vi "RF Streaming to Disk (Host).vi"() -> ()   [LabVIEW 2018]
doc: "This template is for the Simple NI-USRP Streaming design, a design that shows the basics of streaming data to and from an NI USRP-294x/295x device. Refer to the block diagram for more information about how to use this template."
uses:
  <vilib>/userdefined/Silver/nirio_resource_slv.ctl
  typedefs/rx channel config.ctl
  typedefs/rf.channel selector.ctl
  <vilib>/Utility/error.llb/DialogType.ctl
  typedefs/rx config.ctl
  SubVIs/RF Rec Start Trigger.ctl
panel:
  out "size (in bytes)":i64
  out "fifo fullness":dbl(slide) scale=0.0..1.0
  out "HW stoped":bool
  in  "Rec file":path=path "C:/Users/PLM_410/Загрузки/RF Recorder test.bin"
  in  "rf channel selector":T1
  in  "rx channel config":T2={"antenna"="RX2", "frequency"=2000000000.0, "lo frequency"=-1.0, "level"=0.0} {"frequency" format="%#.3pHz"; "lo frequency" format="%#.3pHz"; "level" format="%#_gdBm"}
  in  "number of samples":u32=8192 caption="Number of Samples"
  in  "sample rate":dbl=10000000.0 caption="Sample Rate" format="%#.3pS/s"
  in  "transfer mode":enum16{"Finite", "Continuous"}(ring) caption="Acquisition Mode"
  in  "USRP RIO device":T3="MXI1Port1Dev1" caption="USRP RIO Device"
  in  "indicator tab":T4(tab)
  out "power spectrum":cluster{"f0":dbl, "df":dbl, "magnitude":dbl[]}(graph) caption="Power Spectrum"
  out "power level":dbl[](graph) caption="Power Level"
  out "iq data":waveform(dbl)[](graph) caption="I & Q Data"
  out "rx.coerced configurations":T5 {"coerced sample rates" format="%#.3pS/s"; "coerced levels" format="%#.3gdBm"; "coerced lo frequencies" format="%#.3pHz"; "coerced frequencies" format="%#.3pHz"}
  in  "rx.stop":bool
  # "NI-USRP RIO Streaming to Disk"
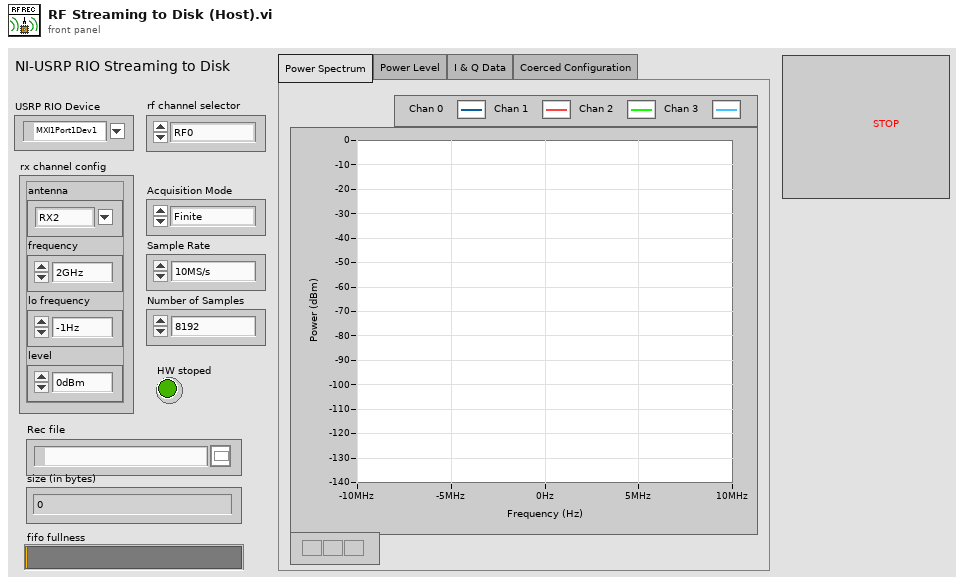
[diagram p1: front panel]
types:
  T1 = typedef "rf.channel selector.ctl" = enum16{"RF0", "RF1"}
  T2 = typedef "rx channel config.ctl" = cluster{"antenna":string, "frequency":dbl, "lo frequency":dbl, "level":dbl}
  T3 = typedef "nirio_resource_slv.ctl" = tag
  T4 = enum32{"Power Spectrum", "Power Level", "I & Q Data", "Coerced Configuration"}
  T5 = cluster{"coerced frequencies":dbl[], "coerced lo frequencies":dbl[], "coerced levels":dbl[], "coerced sample rates":dbl[]}
  T6 = enum16{"open", "replace", "create", "open or create", "replace or create", "replace or create with confirmation"}
  T7 = typedef "RF Rec Start Trigger.ctl" = enum8{"Software", "Digital Edge", "Rx Start Trigger", "Tx Start Trigger", "Immediate", "Future Time Event"}
  T8 = typedef "rx config.ctl" = cluster{"rf enable 0":bool, "rf config 0":cluster{"antenna":string, "frequency":dbl, "lo frequency":dbl, "level":dbl}, "rf enable 1":bool, "rf config 1":cluster{"antenna":string, "frequency":dbl, "lo frequency":dbl, "level":dbl}, "transfer mode":enum16{"Finite", "Continuous"}, "sample rate":dbl, "number of samples":u32, "start trigger":T7}
  T9 = cluster{"daughterboard 0 lo configuration":enum16{"Independent", "Import", "Shared and Export", "Reimport", "Shared"}, "daughterboard 1 lo configuration":enum16{"Independent", "Import", "Shared and Export", "Reimport", "Shared"}}
  T10 = typedef "DialogType.ctl" = u16
  T11 = typedef "niUsrpRio Config v1 Host.lvlib/niUsrpRio Session.ctl" = cluster{"FPGA Interface":refnum<k20>, "RIO Interface Number":u32, "Data Clock Rate":u32, "FPGA Data Clock Rate":u32, "Global Settings Register Bus":T12, "Radio 0 Settings Register Bus":T12, "Radio 1 Settings Register Bus":T12, "Radio Settings Bus Semaphore":T13, "DB Queues":T14[], "Characterization Data Valid?":bool, "EEPROM Header":T15, "Device Data Header":T16, "EEPROM Characterization Header":T17, "Characterization Data":T18[], "FPGA Current Version":u32, "FPGA Oldest Compatible Version":u32, "Fixed Logic Current Version":u32, "Fixed Logic Oldest Compatible Version":u32, "FPGA Radio Settings Bus Current Version":u32, "FPGA Radio Settings Bus Oldest Compatible Version":u32, "FPGA Board Config Current Version":u32, "FPGA Board Config Oldest Compatible Version":u32, "Daughterboard Clock Rate":u32, "daughterboard configuration session handles":u64[]}
  T12 = typedef "niInstr Register Bus v0 Host.lvlib/Register Bus Session.ctl" = refnum<queue>
  T13 = typedef "Semaphore RefNum" = refnum<k1>
  T14 = typedef "niUsrpRio Config v1 Host.lvlib/DB Queue Reference.ctl" = refnum<queue>
  T15 = typedef "niUsrpRio Config v1 Host.lvlib/EEPROM Header.ctl" = cluster{"Checksum":u32, "Product Code":u16, "Hardware Current Version":u16, "Hardware Oldest Compatible Version":u16, "EEPROM Map Current Version":u16, "EEPROM Map Oldest Compatible Version":u16, "User Password":string, "Pointer to Factory Header":u32, "Pointer to User Header":u32, "Recommended Interval":u16, "Number of Reserved Bytes":i32, "Number of Daughterboards":u8, "Daughterboard IDs":u16[], "Daughterboard Serial Numbers":string[]}
  T16 = typedef "niUsrpRio Config v1 Host.lvlib/EEPROM Device Data Header.ctl" = cluster{"Checksum":u32, "Number of Channels":u8, "Number of Gain Settings":u16[], "Pointer to Characterization Data":u32[], "Number of Reserved Bytes":i32, "Number of Frequencies":u16[]}
  T17 = typedef "niUsrpRio Config v1 Host.lvlib/EEPROM Characterization Header.ctl" = cluster{"Checksum":u32, "Date":timestamp, "Temperature":sgl, "Misc. Info":string, "Pointer to Device Data Header":u32, "Number of Reserved Bytes":i32}
  T18 = typedef "niUsrpRio Config v1 Host.lvlib/Characterization Data.ctl" = cluster{"Gains[dB]":dbl[], "Frequencies [Hz]":dbl[], "IQ Imbalance Table":T19[], "Measured Gains[dB]":dbl[][]}
  T19 = typedef "niUsrpRio Config v1 Host.lvlib/IQ Imbalance.ctl" = cluster{"Gain Imbalance [linear]":dbl, "Phase Imbalance [radians]":dbl, "Offset":cdb}
  T20 = cluster{"channel configuration":cluster{"channel enable":bool, "channel configuration":cluster{"antenna":string, "frequency":dbl, "lo frequency":dbl, "level":dbl}}[], "transfer mode":enum16{"Finite", "Continuous"}, "sample rate":dbl, "number of samples":u32, "start trigger":T7}
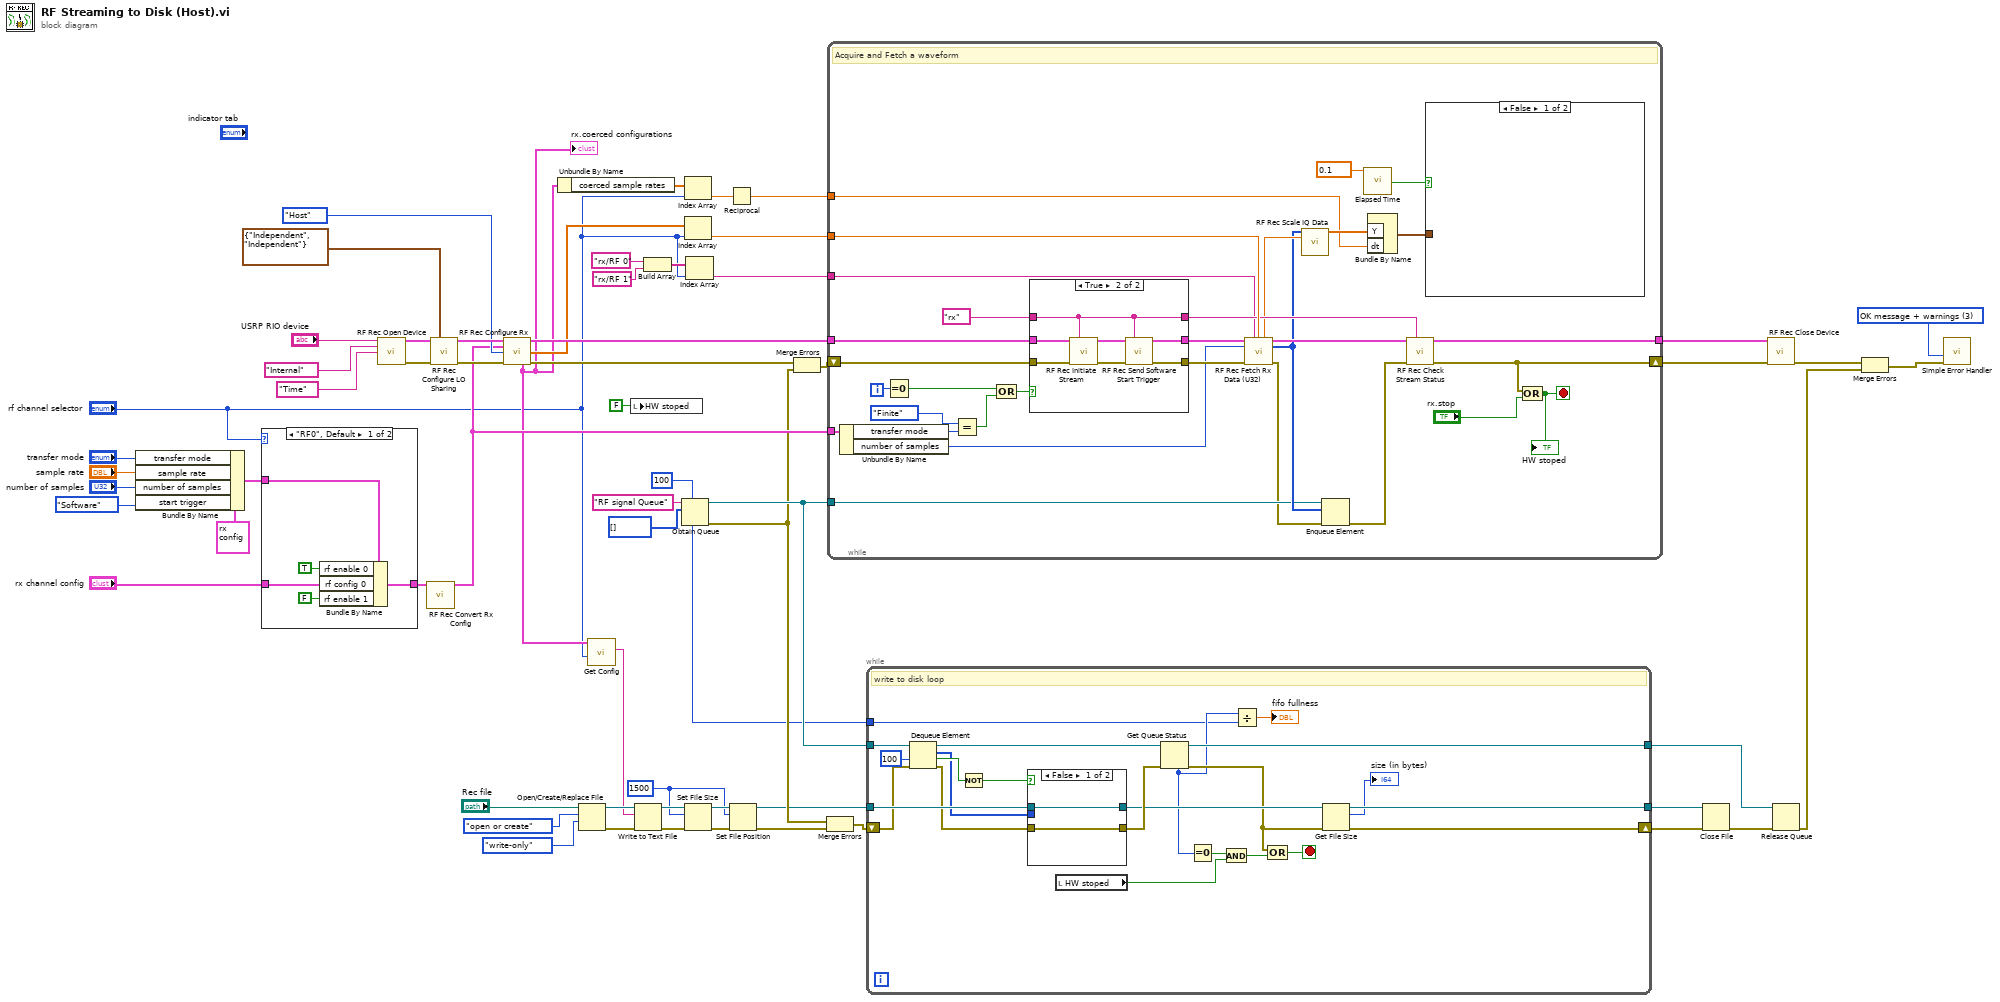
[diagram p0: block diagram]
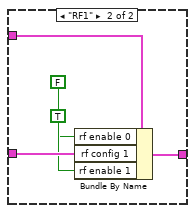
[diagram p2: hidden frame]
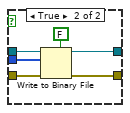
[diagram p3: hidden frame]
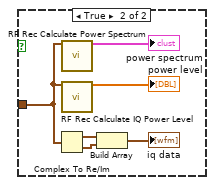
[diagram p5: hidden frame]
diagram:
  w8 = i64 1500 ("size (in bytes)")
  w17 = 100 ("max queue size (-1, unlimited)")
  w62 = T10 3 items=["no dialog", "OK message", "continue or stop message", "OK message + warnings", "continue/stop + warnings"] ("type of dialog (OK msg:1)")
  n1 = Bundle By Name(cluster=T8 {"rf enable 0"=TRUE, "rf config 0"={"antenna"="RX2", "frequency"=2000000000.0, "lo frequency"=-1.0, "level"=0.0}, "rf enable 1"=TRUE, "rf config 1"={"antenna"="RX2", "frequency"=2000000000.0, "lo frequency"=-1.0, "level"=0.0}, "transfer mode"=enum."Finite", "sample rate"=10000000.0, "number of samples"=8192, "start trigger"=enum."Immediate"} ("rx config"), "transfer mode"="transfer mode", "sample rate"="sample rate", "number of samples"="number of samples", "start trigger"=RF_Rec_Start_Trigger."Software") -> (w44:T8)
  n2 = case shown="\"RF0\", Default" "rf channel selector" {
    tunnel: w44 -> [w67 w72]
    tunnel: "rx channel config" -> [w66 w71]
    tunnel: [w63 w68] -> w42
    frame "RF0", Default {
      n3 = Bundle By Name(cluster=w67, "rf enable 0"=TRUE, "rf config 0"=w66, "rf enable 1"=FALSE) -> (w63:T8)
    }
    frame "RF1" {
      n4 = Bundle By Name(cluster=w72, "rf enable 0"=FALSE, "rf config 1"=w71, "rf enable 1"=TRUE) -> (w68:T8)
    }
  }
  n5 = call "RF Rec Open Device.vi"("USRP RIO device"="USRP RIO device", "Reference Frequency Source"="Internal" ("reference frequency source"), "which bitfile"="Time") -> ("niUsrpRio Session (out)"=w55:T11, "error out"=w54:errorcluster)  [unwired: 11 in]
  n6 = call "RF Rec Convert Rx Config.vi"("rx config"=w42) -> ("rx config out"=w41:T20)  [unwired: 14 in]
  n7 = call "RF Rec Configure LO Sharing.vi"("niUsrpRio Session in"=w55, "lo config"=T9 {"daughterboard 0 lo configuration"=enum."Independent", "daughterboard 1 lo configuration"=enum."Independent"}, "error in"=w54) -> ("niUsrpRio Session out"=w53:T11, "error out"=w52:errorcluster)  [unwired: 11 in]
  n8 = call "RF Rec Configure Rx.vi"("niUsrpRio Session"=w53, "rx config"=w41, "rx.data sink"=enum16{"SFP Port 0", "SFP Port 1", "Host"}."Host", "error in"=w52) -> ("niUsrpRio Session (out)"=w40:T11, "vertical range"=w38:dbl[], "rx.coerced configurations"=w15:T5, "error out"=w39:errorcluster)  [unwired: 7 in, 1 out]
  "rx.coerced configurations" <- w15
  n9 = Unbundle By Name(w15) -> ("coerced sample rates"=w36:dbl[])
  n10 = Open/Create/Replace File(file path (use dialog)="Rec file", operation (0:open)=T6."open or create", access (0:read/write)=enum16{"read/write", "read-only", "write-only"}."write-only") -> (refnum out=w16:refnum<file>, error out=w13:errorcluster)  [unwired: 3 in, 1 out]
  n11 = call "Get Config.vi"("rf channel selector"="rf channel selector", "rx.coerced configurations"=w15) -> ("file preamble"=w14:string)  [unwired: 9 in]
  n12 = local write "HW stoped"(FALSE ("HW stoped")) -> ()
  n13 = Write to Text File(file (use dialog)=w16, text=w14, error in=w13) -> (refnum out=w11:refnum<file>, error out=w12:errorcluster)  [unwired: 1 in, 1 out]
  n14 = Build Array("rx/RF 0", "rx/RF 1") -> (w3:string[])
  n15 = Obtain Queue(max queue size (-1, unlimited)=w17, name (unnamed)="RF signal Queue", element data type=u32[] []) -> (queue out=w30:refnum<queue>, error out=w25:errorcluster)  [unwired: 2 in, 1 out]
  n16 = Index Array(array=w36, index="rf channel selector") -> (element=w35:dbl)
  n17 = Index Array(array=w38, index="rf channel selector") -> (element=w37:dbl)
  n18 = Set File Size(4:w12, 6:w8, 7:w11) -> (0:w10:errorcluster, 3:w9:refnum<file>)
  n19 = Index Array(array=w3, index="rf channel selector") -> (element=w1:string)
  n20 = Reciprocal(x=w35) -> (1/x=w34:dbl)
  n21 = Set File Position(offset (in bytes) (0)=w8, refnum=w9, error in=w10) -> (refnum out=w7:refnum<file>, error out=w6:errorcluster)  [unwired: 1 in]
  n22 = Merge Errors(w39, w25) -> (w31:errorcluster)
  n23 = Merge Errors(w25, w6) -> (w26:errorcluster)
  n24 = while {
    tunnel: [w85] -> w59
    shift-right: [w84] -> w60
    shift-left: w31 -> [w98]
    tunnel: w41 -> [w97]
    tunnel: w40 -> [w91]
    tunnel: w37 -> [w87]
    tunnel: w34 -> [w78]
    tunnel: w30 -> [w76]
    tunnel: w1 -> [w73]
    i -> [w102]
    stop <- w101 stop-if-true
    # "Acquire and Fetch a waveform"
    n25 = Unbundle By Name(w97) -> ("transfer mode"=w96:enum16{"Finite", "Continuous"}, "number of samples"=w88:u32)
    n26 = Equal To 0?(x=w102) -> (x = 0?=w94:bool)
    n27 = Equal?(x=enum16{"Finite", "Continuous"}."Finite" ("y"), y=w96) -> (x = y?=w93:bool)
    n28 = Compound Arithmetic op=OR(w94, w93) -> (w92:bool)
    n29 = case shown="True" w92 {
      tunnel: w98 -> [w105 w113]
      tunnel: w91 -> [w106 w110]
      tunnel: [w106 w109] -> w90
      tunnel: [w105 w108] -> w89
      tunnel: "rx" ("scope") -> [w104 w107]
      tunnel: [w104 w107] -> w82
      frame False {
      }
      frame True {
        n30 = call "RF Rec Initiate Stream.vi"("niUsrpRio Session"=w110, "scope"=w107, "error in"=w113) -> ("niUsrpRio Session (out)"=w112:T11, "error out"=w111:errorcluster)  [unwired: 11 in]
        n31 = call "RF Rec Send Software Start Trigger.vi"("niUsrpRio Session"=w112, "scope"=w107, "error in"=w111) -> ("niUsrpRio Session (out)"=w109:T11, "error out"=w108:errorcluster)  [unwired: 11 in]
      }
    }
    n32 = call "RF Rec Fetch Rx Data (U32).vi"("niUsrpRio Session"=w90, "scope"=w73, "vertical range"=w87, "number of samples"=w88, "error in"=w89) -> ("scaling (V/code)"=w81:dbl, "niUsrpRio Session (out)"=w86:T11, "waveform data"=w77:u32[], "error out"=w75:errorcluster)  [unwired: 7 in]
    n33 = call "RF Rec Scale IQ Data.vi"("raw waveform data"=w77, "scaling (V/code)"=w81) -> ("scaled data"=w80:cdb[])  [unwired: 13 in]
    n34 = Enqueue Element(queue=w76, element=w77, error in (no error)=w75) -> (error out=w74:errorcluster)  [unwired: 1 in, 2 out]
    n35 = call "Elapsed Time"("Time Target (s)"=0.1 ("retrigger delay")) -> ("Time has Elapsed"=w100:bool)  [unwired: 11 in, 7 out]
    n36 = Bundle By Name("Y"=w80, "dt"=w78) -> (w79:waveform(cdb))  [unwired: 1 in]
    n37 = call "RF Rec Check Stream Status.vi"("niUsrpRio Session"=w86, "scope"=w82, "error in"=w74) -> ("niUsrpRio Session (out)"=w85:T11, "error out"=w84:errorcluster)  [unwired: 10 in, 1 out]
    n38 = case shown="False" w100 {
      tunnel: w79 -> [_ w119]
      frame False {
      }
      frame True {
        n39 = Complex To Re/Im(x + iy=w119) -> (x=w115:waveform(dbl), y=w114:waveform(dbl))
        n40 = call "RF Rec Calculate Power Spectrum.vi"("waveform"=w119) -> ("power spectrum (dBm)"=→"power spectrum":cluster{"f0":dbl, "df":dbl, "magnitude":dbl[]})  [unwired: 14 in]
        n41 = call "RF Rec Calculate IQ Power Level.vi"("iq data"=w119) -> ("power level (dBm)"=→"power level":dbl[])  [unwired: 14 in]
        n42 = Build Array(w115, w114) -> (→"iq data":waveform(dbl)[])
      }
    }
    n43 = Compound Arithmetic op=OR(w84, "rx.stop") -> (w101:bool)
    "HW stoped" <- w101
  }
  n44 = while {
    tunnel: w30 -> [w141]
    tunnel: w7 -> [w142]
    tunnel: [w124] -> w24
    shift-right: [w125] -> w23
    shift-left: w26 -> [w140]
    tunnel: [w132] -> w22
    tunnel: w17 -> [w122]
    stop <- w130 stop-if-true
    # "write to disk loop"
    n45 = Dequeue Element(queue=w141, timeout in ms (-1)=100, error in (no error)=w140) -> (queue out=w136:refnum<queue>, element=w135:u32[], timed out?=w138:bool, error out=w134:errorcluster)
    n46 = Not(x=w138) -> (.not. x?=w137:bool)
    n47 = case shown="False" w137 {
      tunnel: w142 -> [w144 w150]
      tunnel: w135 -> [_ w149]
      tunnel: w134 -> [w143 w148]
      tunnel: [w144 w146] -> w127
      tunnel: [w143 w145] -> w133
      frame False {
      }
      frame True {
        n48 = Write to Binary File(file (use dialog)=w150, data=w149, error in=w148, 5:FALSE ("prepend array or string size? (T)")) -> (refnum out=w146:refnum<file>, error out=w145:errorcluster)  [unwired: 2 in, 1 out]
      }
    }
    n49 = local read "HW stoped"() -> (w131:bool)
    n50 = Get Queue Status(queue=w136, error in (no error)=w133) -> (queue out=w132:refnum<queue>, error out=w126:errorcluster, # elements in queue=w123:i32)  [unwired: 1 in, 5 out]
    n51 = Equal To 0?(x=w123) -> (x = 0?=w128:bool)
    n52 = Compound Arithmetic op=AND(w128, w131) -> (w129:bool)
    n53 = Divide(x=w123, y=w122) -> (x/y=→"fifo fullness":dbl)
    n54 = Compound Arithmetic op=OR(w126, w129) -> (w130:bool)
    n55 = Get File Size(file=w127, error in=w126) -> (refnum out=w124:refnum<file>, size (in bytes)=→"size (in bytes)":i64, 0:w125:errorcluster)
  }
  n56 = Close File(refnum=w24, error in=w23) -> (error out=w21:errorcluster)  [unwired: 1 out]
  n57 = call "RF Rec Close Device.vi"("niUsrpRio Session"=w59, "error in"=w60) -> ("error out"=w61:errorcluster)  [unwired: 13 in]
  n58 = Release Queue(queue=w22, error in (no error)=w21) -> (error out=w18:errorcluster)  [unwired: 1 in, 2 out]
  n59 = Merge Errors(w61, w18) -> (w19:errorcluster)
  n60 = call <vilib>:"Simple Error Handler.vi"("type of dialog (OK msg:1)"=w62, "error in (no error)"=w19) -> ()  [unwired: 3 in, 5 out]
